vi "PAN_parseCmds.vi"(7 "Cmd Option":string, 11 "error in":errorcluster, 12 "Modules":string[](array[string])) -> (4 "ImmedReplyString":string, 15 "error out":errorcluster)   [LabVIEW 2016]
doc: "API for the ArcVIEW application. It will receive commands as any other Module API (starting dinamically)"
uses:
  <vilib>/Utility/error.llb/DialogType.ctl
  PAN_Scheduler_action.ctl
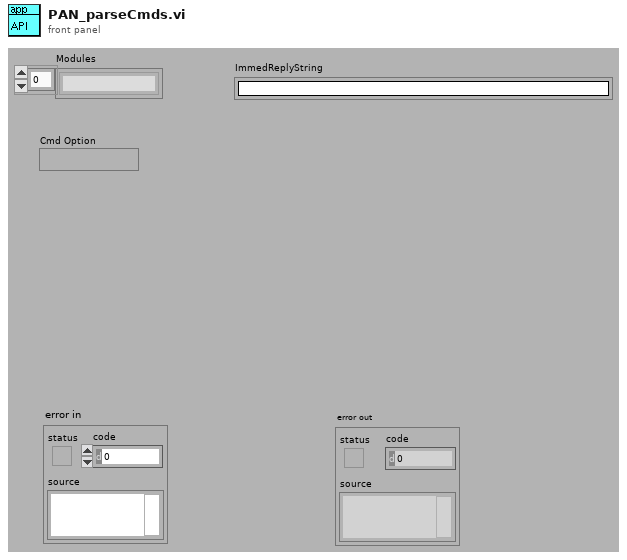
[diagram p1: front panel]
types:
  T1 = typedef "PAN_Scheduler_action.ctl" = enum16{"add", "search", "clean", "get all"}
  T2 = typedef "DialogType.ctl" = u16
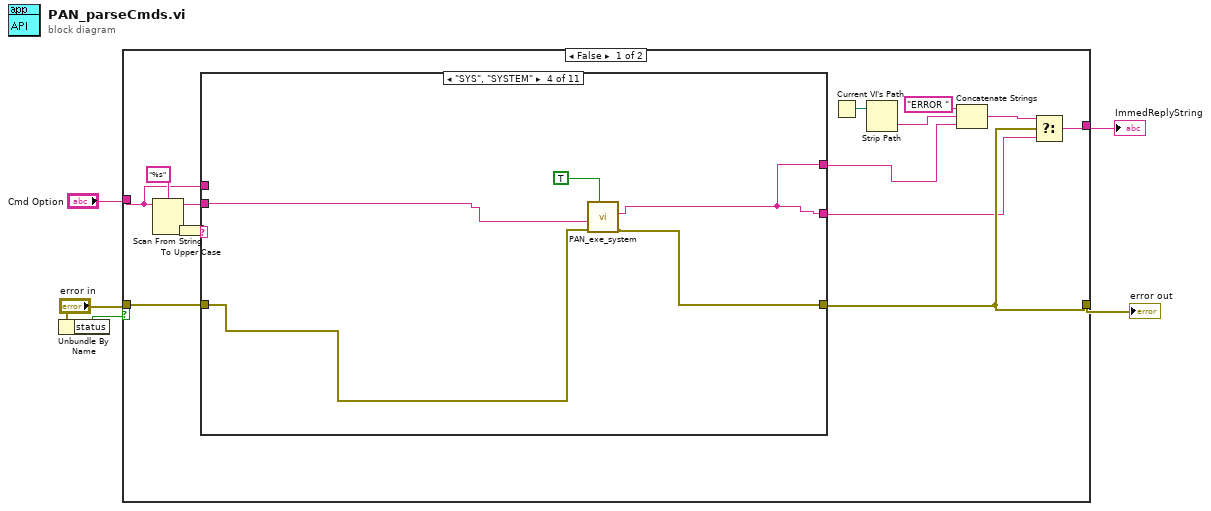
[diagram p0: block diagram]
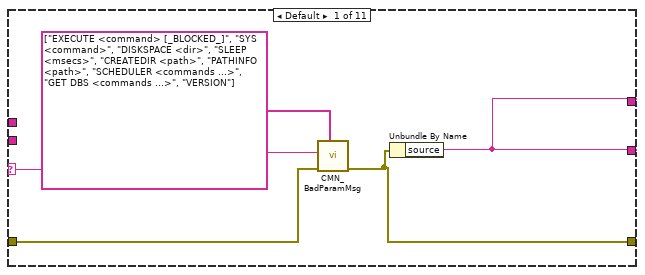
[diagram p2: hidden frame]
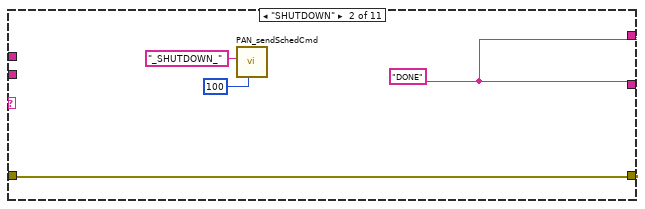
[diagram p3: hidden frame]
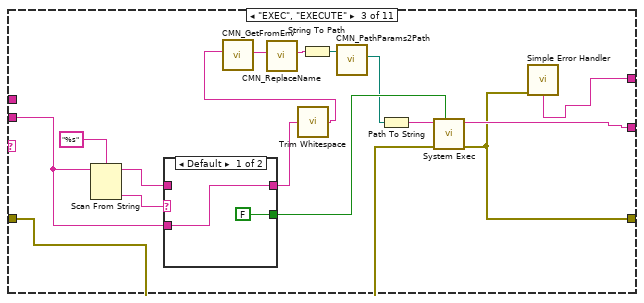
[diagram p4: hidden frame]
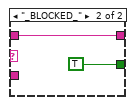
[diagram p5: hidden frame]
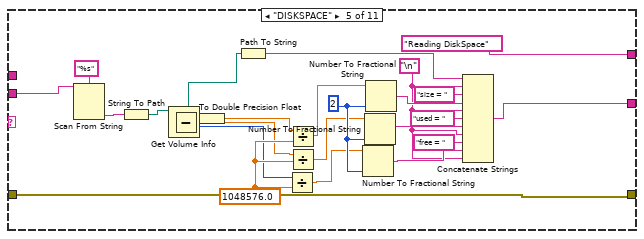
[diagram p6: hidden frame]
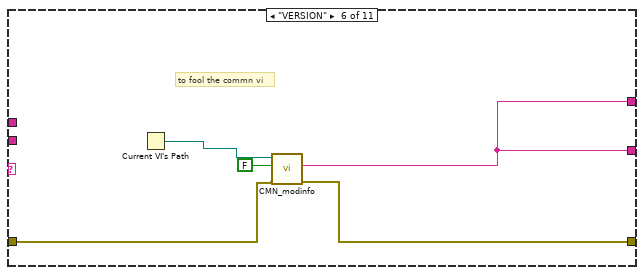
[diagram p7: hidden frame]
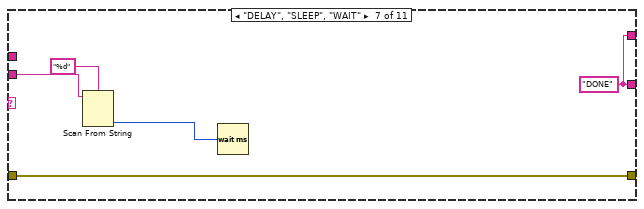
[diagram p8: hidden frame]
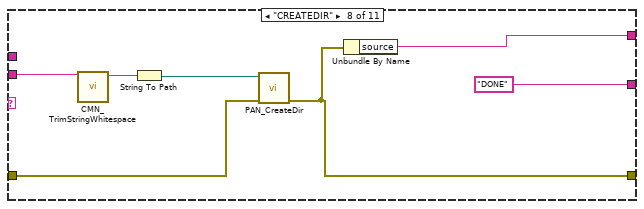
[diagram p9: hidden frame]
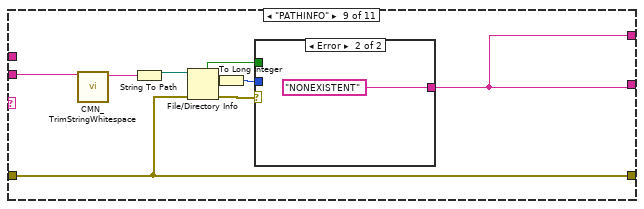
[diagram p10: hidden frame]
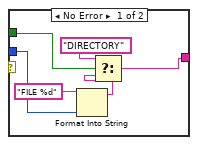
[diagram p11: hidden frame]
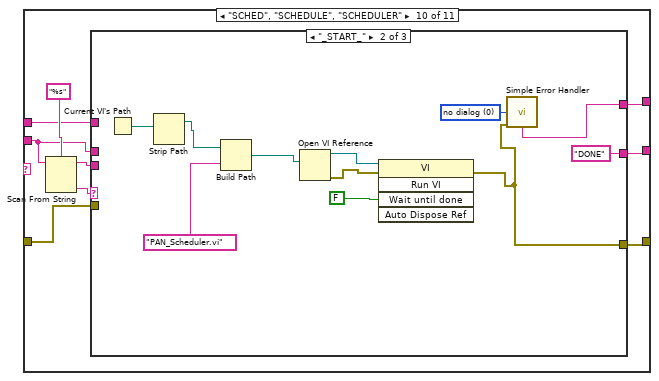
[diagram p12: hidden frame]
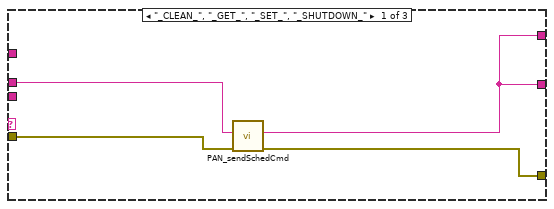
[diagram p13: hidden frame]
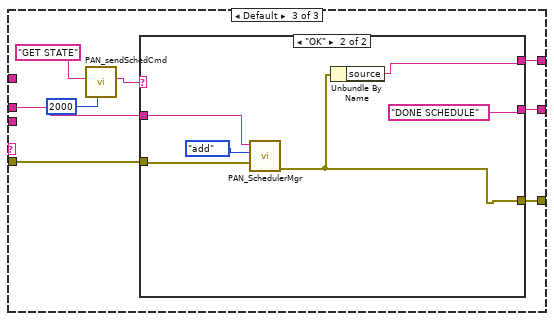
[diagram p14: hidden frame]
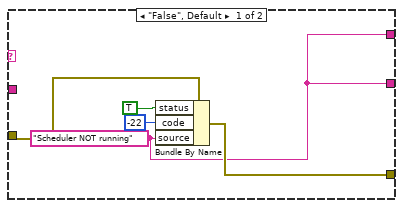
[diagram p15: hidden frame]
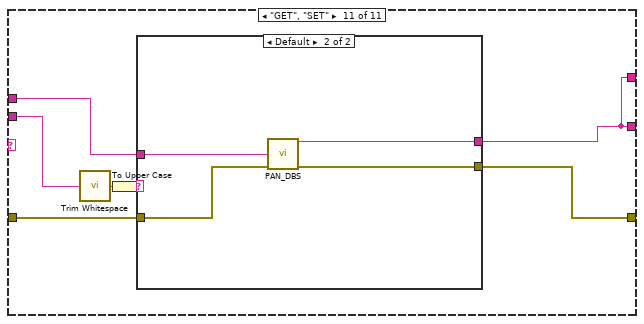
[diagram p16: hidden frame]
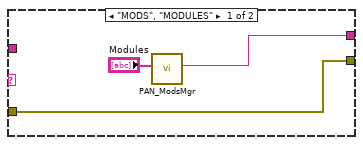
[diagram p17: hidden frame]
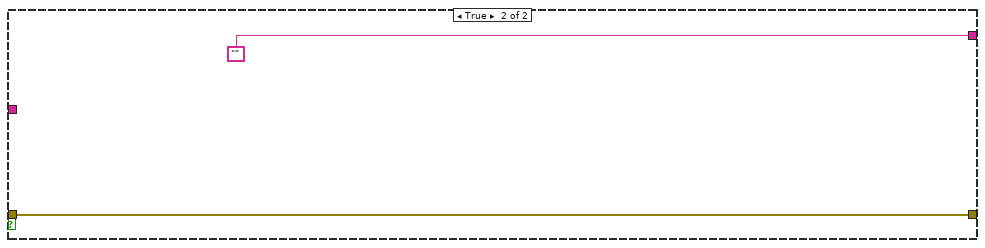
[diagram p18: hidden frame]
diagram:
  n1 = Unbundle By Name("error in") -> ("status"=w3:bool)
  n2 = case shown="False" w3 {
    tunnel: "error in" -> [w19 w170]
    tunnel: [w12 w170] -> w1
    tunnel: [w11 ""] -> w5
    tunnel: "Cmd Option" -> [w8 _]
    frame False {
      n3 = Scan From String(format string="%s" ("Format String"), input string=w8) -> (remaining string=w7:string, output 1=w18:string)  [unwired: 2 in, 3 out]
      n4 = To Upper Case(1:w18) -> (0:w6:string)
      n5 = case shown="\"SYS\", \"SYSTEM\"" w6 {
        selector: w6 -> [w24 _ _ _ _ _ _ _ _ _ _]
        tunnel: w19 -> [w23 w28 w39 w53 w64 w82 w85 w92 w100 w120 w160]
        tunnel: [w22 w28 w37 w52 w64 w81 w85 w90 w100 w119 w161] -> w12
        tunnel: [w21 w27 w36 w50 "Reading DiskSpace" ("message") w80 w84 w89 w99 w117 w159] -> w10
        tunnel: [w21 w27 w38 w50 w65 w80 w84 "DONE" w99 w118 w159] -> w9
        tunnel: w8 -> [_ _ _ _ _ _ _ _ _ w112 w158]
        tunnel: w7 -> [_ _ w40 w51 w55 _ w88 w95 w104 w115 w157]
        frame Default {
          n6 = call "CMN_BadParamMsg.vi"("valid params"=string[] ["EXECUTE <command> [_BLOCKED_]", "SYS <command>", "DISKSPACE <dir>", "SLEEP <msecs>", "CREATEDIR <path>", "PATHINFO <path>", "SCHEDULER <commands ...>", "GET DBS <commands ...>", "VERSION"], "error in (no error)"=w23, "parameter"=w24) -> ("error out"=w22:errorcluster)  [unwired: 1 in, 7 out]
          n7 = Unbundle By Name(w22) -> ("source"=w21:string)
        }
        frame "SHUTDOWN" {
          w27 = "DONE"
          n8 = call "PAN_sendSchedCmd.vi"("timeout in ms (5000)"=100, "command"="_SHUTDOWN_") -> ()  [unwired: 1 in, 9 out]
        }
        frame "EXEC", "EXECUTE" {
          n9 = Scan From String(format string="%s", input string=w40) -> (remaining string=w43:string, output 1=w35:string)  [unwired: 2 in, 3 out]
          n10 = case shown="Default" w35 {
            tunnel: w43 -> [_ w48]
            tunnel: [w46 w48] -> w42
            tunnel: [FALSE TRUE] -> w41
            tunnel: w40 -> [w46 _]
            frame Default {
            }
            frame "_BLOCKED_" {
            }
          }
          n11 = call <vilib>:"Trim Whitespace.vi"("string"=w42) -> ("trimmed string"=w31:string)  [unwired: 1 in]
          n12 = call "CMN_GetFromEnv.vi"("str in"=w31) -> ("str out"=w32:string)  [unwired: 10 out]
          n13 = call "CMN_ReplaceName.vi"("name in"=w32) -> ("name out"=w34:string)  [unwired: 1 in, 9 out]
          n14 = String To Path(string=w34) -> (path=w33:path)
          n15 = call "CMN_PathParams2Path.vi"("Path In"=w33) -> ("Path out"=w30:path)  [unwired: 2 in, 8 out]
          n16 = Path To String(path=w30) -> (string=w29:string)
          n17 = call <vilib>:"System Exec.vi"("wait until completion? (T)"=w41, "error in (no error)"=w39, "command line"=w29) -> ("error out"=w37:errorcluster, "standard output"=w38:string)  [unwired: 3 in, 4 out]
          n18 = call <vilib>:"Simple Error Handler.vi"("error in (no error)"=w37) -> ("message"=w36:string)  [unwired: 1 in, 7 out]
        }
        frame "SYS", "SYSTEM" {
          n19 = call "PAN_exe_system.vi"("wait until completion? (T)"=TRUE, "error in (no error)"=w53, "command line"=w51) -> ("error out"=w52:errorcluster, "response"=w50:string)  [unwired: 1 in, 6 out]
        }
        frame "DISKSPACE" {
          w73 = sgl 1048576.0
          w74 = i16 2 ("precision (6)")
          w56 = "\n"
          n20 = Scan From String(format string="%s" ("Format String"), input string=w55) -> (output 1=w77:string)  [unwired: 2 in, 4 out]
          n21 = String To Path(string=w77) -> (path=w66:path)
          n22 = Get Volume Info(11:w66) -> (1:w70:i64, 2:w54:i64, 5:w76:path)  [unwired: 1 in, 3 out]
          n23 = To Double Precision Float(number=w54) -> (double precision float=w72:dbl)
          n24 = Subtract(x=w72, y=w70) -> (x-y=w71:dbl)
          n25 = Path To String(path=w76) -> (string=w75:string)
          n26 = Divide(x=w70, y=w73) -> (x/y=w67:sgl)
          n27 = Divide(x=w72, y=w73) -> (x/y=w69:dbl)
          n28 = Divide(x=w71, y=w73) -> (x/y=w68:dbl)
          n29 = Number To Fractional String(number=w67, precision (6)=w74) -> (F-format string=w57:string)  [unwired: 2 out]
          n30 = Number To Fractional String(number=w68, precision (6)=w74) -> (F-format string=w59:string)  [unwired: 2 out]
          n31 = Number To Fractional String(number=w69, precision (6)=w74) -> (F-format string=w61:string)  [unwired: 2 out]
          n32 = Concatenate Strings(w75, w56, "size = " ("string"), w61, w56, "used = " ("string"), w59, w56, "free = " ("string"), w57, w56) -> (w65:string)
        }
        frame "VERSION" {
          # "to fool the commn vi"
          n33 = Current VI's Path() -> (path=w79:path)
          n34 = call "CMN_modinfo.vi"("error in (no error)"=w82, "full"=FALSE, "caller path"=w79) -> ("error out"=w81:errorcluster, "INFO"=w80:string)  [unwired: 7 out]
        }
        frame "DELAY", "SLEEP", "WAIT" {
          w84 = "DONE" ("value")
          n35 = Scan From String(format string="%d", input string=w88) -> (output 1=w86:i32)  [unwired: 2 in, 4 out]
          n36 = Wait (ms)(milliseconds to wait=w86) -> ()  [unwired: 1 out]
        }
        frame "CREATEDIR" {
          n37 = call "CMN_TrimStringWhitespace.vi"("string"=w95) -> ("trimmed string"=w94:string)  [unwired: 1 in, 8 out]
          n38 = String To Path(string=w94) -> (path=w93:path)
          n39 = call "PAN_CreateDir.vi"("error in"=w92, "dir to create"=w93) -> ("error"=w90:errorcluster)  [unwired: 8 out]
          n40 = Unbundle By Name(w90) -> ("source"=w89:string)
        }
        frame "PATHINFO" {
          n41 = call "CMN_TrimStringWhitespace.vi"("string"=w104) -> ("trimmed string"=w103:string)  [unwired: 1 in, 8 out]
          n42 = String To Path(string=w103) -> (path=w102:path)
          n43 = File/Directory Info(path=w102, error in=w100) -> (directory=w98:bool, size=w96:i64, error out=w101:errorcluster)  [unwired: 4 out]
          n44 = To Long Integer(number=w96) -> (32bit integer=w97:i32)
          n45 = case shown="Error" w101 {
            tunnel: [w108 "NONEXISTENT"] -> w99
            tunnel: w98 -> [w110 _]
            tunnel: w97 -> [w107 _]
            frame No Error {
              n46 = Format Into String(format string="FILE %d" ("f"), w107) -> (resulting string=w105:string)  [unwired: 2 in, 1 out]
              n47 = Select(t="DIRECTORY", s=w110, f=w105) -> (s? t:f=w108:string)
            }
            frame Error {
            }
          }
        }
        frame "SCHED", "SCHEDULE", "SCHEDULER" {
          n48 = Scan From String(format string="%s", input string=w115) -> (remaining string=w113:string, output 1=w114:string)  [unwired: 2 in, 3 out]
          n49 = case shown="\"_START_\"" w114 {
            tunnel: w120 -> [w124 _ w143]
            tunnel: [w122 "DONE" w142] -> w118
            tunnel: [w123 w131 w141] -> w119
            tunnel: [w122 w134 w140] -> w117
            tunnel: w115 -> [w121 _ w139]
            tunnel: w113 -> [_ _ _]
            tunnel: w112 -> [_ _ _]
            frame "_CLEAN_", "_GET_", "_SET_", "_SHUTDOWN_" {
              n50 = call "PAN_sendSchedCmd.vi"("error in (no error)"=w124, "command"=w121) -> ("error out"=w123:errorcluster, "response"=w122:string)  [unwired: 1 in, 7 out]
            }
            frame "_START_" {
              w135 = T2 0 items=["no dialog", "OK message", "continue or stop message", "OK message + warnings", "continue/stop + warnings"] ("type of dialog (OK msg:1)")
              n51 = Current VI's Path() -> (path=w133:path)
              n52 = Strip Path(path=w133) -> (stripped path=w127:path)  [unwired: 1 out]
              n53 = Build Path(base path=w127, name or relative path="PAN_Scheduler.vi") -> (appended path=w126:path)
              n54 = Open VI Reference(vi path=w126) -> (vi reference=w129:refnum<vi>, error out=w132:errorcluster)  [unwired: 1 in, 4 out]
              n55 = invoke class="VI" method="Run VI"(reference=w129, error in=w132, "Wait until done"=FALSE) -> (error out=w131:errorcluster)  [unwired: 2 in, 4 out]
              n56 = call <vilib>:"Simple Error Handler.vi"("type of dialog (OK msg:1)"=w135, "error in (no error)"=w131) -> ("message"=w134:string)  [unwired: 7 out]
            }
            frame Default {
              n57 = call "PAN_sendSchedCmd.vi"("timeout in ms (5000)"=2000, "command"="GET STATE") -> ("response"=w137:string)  [unwired: 1 in, 8 out]
              n58 = case shown="\"OK\"" w137 {
                tunnel: w143 -> [w148 w153]
                tunnel: [w144 "DONE SCHEDULE"] -> w142
                tunnel: [w147 w151] -> w141
                tunnel: [w144 w150] -> w140
                tunnel: w139 -> [_ w149]
                frame "False", Default {
                  w144 = "Scheduler NOT running" ("source")
                  n59 = Bundle By Name(cluster=w148, "status"=TRUE, "code"=-22, "source"=w144) -> (w147:errorcluster)
                }
                frame "OK" {
                  n60 = call "PAN_SchedulerMgr.vi"("error in (no error)"=w153, "action"=PAN_Scheduler_action."add", "command"=w149) -> ("error out"=w151:errorcluster)  [unwired: 8 out]
                  n61 = Unbundle By Name(w151) -> ("source"=w150:string)
                }
              }
            }
          }
        }
        frame "GET", "SET" {
          n62 = call <vilib>:"Trim Whitespace.vi"("string"=w157) -> ("trimmed string"=w156:string)  [unwired: 1 in]
          n63 = To Upper Case(1:w156) -> (0:w155:string)
          n64 = case shown="Default" w155 {
            tunnel: [w163 w168] -> w161
            tunnel: w160 -> [w163 w167]
            tunnel: [w164 w166] -> w159
            tunnel: w158 -> [_ w165]
            frame "MODS", "MODULES" {
              n65 = call "PAN_ModsMgr.vi"("Modules"="Modules") -> ("response"=w164:string)  [unwired: 10 out]
            }
            frame Default {
              n66 = call "PAN_DBS.vi"("Cmd"=w165, "error in"=w167) -> ("ImmedReplyString"=w166:string, "error out"=w168:errorcluster)  [unwired: 12 out]
            }
          }
        }
      }
      n67 = Current VI's Path() -> (path=w15:path)
      n68 = Strip Path(path=w15) -> (name=w14:string)  [unwired: 1 out]
      n69 = Concatenate Strings("ERROR ", w14, w10) -> (w13:string)
      n70 = Select(t=w13, s=w12, f=w9) -> (s? t:f=w11:string)
    }
    frame True {
    }
  }
  "error out" <- w1
  "ImmedReplyString" <- w5
